vi "Get Sections.vi"(11 "Object Dictionary in":refnum<class "Object Dictionary.lvclass">) -> (2 "OD Sections":refnum<class "OD Section.lvclass">[](array[class]), 3 "Object Dictionary out":refnum<class "Object Dictionary.lvclass">)   [LabVIEW 2024, in "EDS.lvlib" / "Object Dictionary.lvclass"]
uses:
  Object Dictionary.lvclass
  Object Dictionary.lvclass/Object Dictionary.ctl
  OD Section/OD Section.lvclass
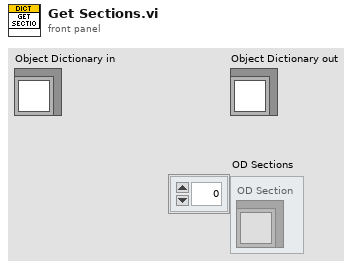
[diagram p1: front panel]
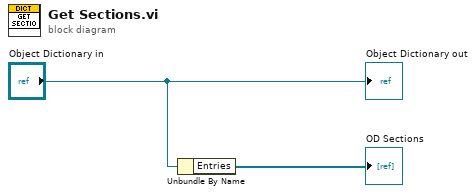
[diagram p0: block diagram]
diagram:
  n1 = Unbundle By Name("Object Dictionary in") -> ("Entries"=→"OD Sections":refnum<class "OD Section.lvclass">[])
  "Object Dictionary out" <- "Object Dictionary in"
